vi "get_idn.vi"(0 "HGF_DeviceBase":refnum<class "HGF_DeviceBase.lvclass">, 5 "error in (no error)":errorcluster) -> (14 "dup HGF_DeviceBase":refnum<class "HGF_DeviceBase.lvclass">, 15 "driverRevision":string="unknown", 16 "firmwareRevision":string="unknown", 17 "vendor":string="unknown", 18 "model":string="unknown", 19 "error out":errorcluster)   [LabVIEW 2014, in "HGF_DeviceBaseClasses.lvlib" / "HGF_DeviceBase.lvclass"]
doc: "Read instrument driver revision, firmware revision, vendor, model, etc."
uses:
  HGF_DeviceBase.lvclass
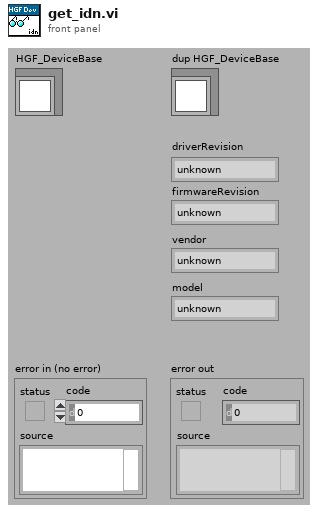
[diagram p1: front panel]
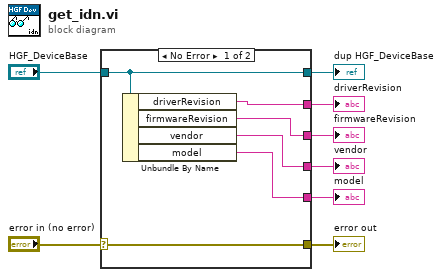
[diagram p0: block diagram]
diagram:
  n1 = case shown="No Error" "error in (no error)" {
    selector: "error in (no error)" -> [w14 w15]
    tunnel: [w14 w15] -> w7
    tunnel: [w13 w16] -> w5
    tunnel: "HGF_DeviceBase" -> [w13 w16]
    tunnel: [w12 _] -> w4
    tunnel: [w11 _] -> w3
    tunnel: [w10 _] -> w2
    tunnel: [w9 _] -> w1
    frame No Error {
      n2 = Unbundle By Name(w13) -> ("driverRevision"=w12:string, "firmwareRevision"=w11:string, "vendor"=w10:string, "model"=w9:string)
    }
    frame Error {
    }
  }
  "error out" <- w7
  "dup HGF_DeviceBase" <- w5
  "driverRevision" <- w4
  "firmwareRevision" <- w3
  "vendor" <- w2
  "model" <- w1
